vi "ScrimCode.vi"() -> ()   [LabVIEW 2017]
uses:
  050-Tests/Wall Following/XY.ctl
  040-typeDefs/LidarPoint.ctl
  <vilib>/myRIO/Common/Instrument Driver Framework/myRIO v1.0/Encoder/typedefs/Encoder Signal Mode.ctl
  <vilib>/myRIO/Instrument Drivers/Onboard IO/Encoder/typedefs/Encoder Reference.ctl
  <vilib>/myRIO/Common/Instrument Driver Framework/Utilities/typedefs/myRIO Generic Hardware Reference.ctl
  <vilib>/myRIO/Common/Instrument Driver Framework/Utilities/typedefs/Hardware Version Enum.ctl
  <vilib>/myRIO/Common/Instrument Driver Framework/Utilities/typedefs/myRIO v1.0 Reference.ctl
  <vilib>/myRIO/Common/Instrument Driver Framework/Utilities/typedefs/Generic FPGA Reference.ctl
  <vilib>/myRIO/Common/Instrument Driver Framework/myRIO v1.0/Encoder/typedefs/Encoder Channels Enum.ctl
  <vilib>/myRIO/Common/Instrument Driver Framework/myRIO v1.0/Encoder/typedefs/Encoder Configuration v1.0.ctl
  <vilib>/userdefined/High Color/nirio_resource_hc.ctl
  <vilib>/myRIO/Common/Instrument Driver Framework/Utilities/vis/Is FPGA Ref Available.vi
  <vilib>/myRIO/Common/Instrument Driver Framework/myRIO v1.0/Encoder/vis/myRIO v1.1 Open Encoder.vi
  <vilib>/myRIO/Instrument Drivers/Onboard IO/Encoder/vis/Read.vi
  <vilib>/myRIO/Common/Instrument Driver Framework/Utilities/vis/Validate Channels.vi
  <vilib>/myRIO/Common/Instrument Driver Framework/myRIO v1.0/Encoder/vis/myRIO v1.0 Reserve Encoder.vi
  <vilib>/myRIO/Common/Instrument Driver Framework/myRIO v1.0/Encoder/vis/myRIO v1.0 Build MUX Configuration Encoder.vi
  <vilib>/myRIO/Common/Instrument Driver Framework/myRIO v1.0/Resource Manager/vis/myRIO v1.0 Reserve Channel List.vi
  <vilib>/myRIO/Common/Instrument Driver Framework/myRIO v1.0/Resource Manager/vis/myRIO v1.0 Create Configuration List.vi
  <vilib>/myRIO/Common/Instrument Driver Framework/myRIO v1.0/Resource Manager/vis/myRIO v1.0 Reserve Channel.vi
  <vilib>/myRIO/Common/Instrument Driver Framework/myRIO v1.0/Resource Manager/vis/myRIO v1.0 Unreserve Channel.vi
  <vilib>/myRIO/Common/Instrument Driver Framework/myRIO v1.0/Resource Manager/vis/myRIO v1.0 Build Mutex Name.vi
  <vilib>/Utility/VariantDataType/GetNumericInfo.vi
  <vilib>/Utility/error.llb/Error Cluster From Error Code.vi
  <vilib>/myRIO/Common/Instrument Driver Framework/myRIO v1.0/myRIO v1.1 Open.vi
  <vilib>/myRIO/Common/Instrument Driver Framework/Utilities/vis/IO Manager.vi
  <vilib>/myRIO/Common/Instrument Driver Framework/Utilities/vis/Configuration Manager.vi
  <vilib>/myRIO/Common/Instrument Driver Framework/myRIO v1.0/Resource Manager/vis/myRIO v1.0 Configure IO.vi
  <vilib>/myRIO/Common/Instrument Driver Framework/myRIO v1.0/myRIO v1.0 Close.vi
  <vilib>/myRIO/Common/Instrument Driver Framework/myRIO v1.0/Encoder/vis/myRIO v1.0 Configure Encoder.vi
  <vilib>/myRIO/Common/Instrument Driver Framework/myRIO v1.0/Encoder/vis/myRIO v1.0 Read Encoder.vi
  <vilib>/addons/control/pid/pid.llb/PID (DBL).vi
  <vilib>/myRIO/Express VI/Onboard IO/Encoder/Encoder Express VI.xnode
  <vilib>/myRIO/Instrument Drivers/Onboard IO/Encoder/vis/myRIO Encoder Open.xnode
  <vilib>/myRIO/Common/Instrument Driver Framework/myRIO v1.0/Encoder/typedefs/Encoder Count Direction Enum.ctl
  <vilib>/addons/control/pid/NI_PID_pid.lvlib
  <vilib>/myRIO/Instrument Drivers/Onboard IO/Encoder/Encoder.lvlib
panel:
  out "XY Graph":cluster{dbl[], dbl[]}(graph)
  in  "Stop Lidar":bool
  out "LidarXY":T1=[{"X"=0.0, "Y"=-0.0}, {"X"=0.0, "Y"=-0.0}, {"X"=0.0, "Y"=-0.0}, {"X"=0.0, "Y"=-0.0}, {"X"=0.0, "Y"=-0.0}, {"X"=0.0, "Y"=-0.0}, {"X"=0.0, "Y"=-0.0}, {"X"=0.0, "Y"=-0.0}, {"X"=0.0, "Y"=-0.0}, {"X"=0.0, "Y"=-0.0}, {"X"=0.0, "Y"=-0.0}, {"X"=0.0, "Y"=-0.0}, {"X"=0.0, "Y"=-0.0}, {"X"=0.0, "Y"=-0.0}, {"X"=0.0, "Y"=-0.0}, {"X"=0.0, "Y"=-0.0}, {"X"=0.0, "Y"=-0.0}, {"X"=0.0, "Y"=-0.0}, {"X"=0.0, "Y"=-0.0}, {"X"=0.0, "Y"=-0.0}, {"X"=0.0, "Y"=-0.0}, {"X"=0.0, "Y"=-0.0}, {"X"=0.0, "Y"=-0.0}, {"X"=0.0, "Y"=-0.0}, {"X"=0.0, "Y"=-0.0}, {"X"=0.0, "Y"=-0.0}, {"X"=0.0, "Y"=-0.0}, {"X"=0.0, "Y"=-0.0}, {"X"=0.0, "Y"=-0.0}, {"X"=0.0, "Y"=-0.0}, {"X"=0.0, "Y"=-0.0}, {"X"=0.0, "Y"=-0.0}, {"X"=0.0, "Y"=-0.0}, {"X"=0.0, "Y"=-0.0}, {"X"=1175.808659612749, "Y"=-52.94332799957733}, {"X"=1168.1174194020048, "Y"=-45.41689652101715}, {"X"=1160.3783860600606, "Y"=-37.98685515608209}, {"X"=1168.5867974931368, "Y"=-31.07887907782929}, {"X"=1168.7554955939645, "Y"=-23.907980234770854}, {"X"=1168.8801907109664, "Y"=-16.736181269769418}, {"X"=1176.960610420781, "Y"=-9.629201313834}, {"X"=1176.9975381384256, "Y"=-2.4073255047001396}, {"X"=1193.9900103325547, "Y"=4.884181207324338}, {"X"=1195.9374604543593, "Y"=12.230726960306109}, {"X"=1201.8390977672932, "Y"=19.66680141503711}, {"X"=1204.6950410270608, "Y"=27.108266724527297}, {"X"=1207.5047999843382, "Y"=34.58551741384792}, {"X"=1227.2577678305224, "Y"=42.689241029135935}, {"X"=1235.9651999305015, "Y"=50.586802238878725}, {"X"=1235.6315384515906, "Y"=58.169589853765174}, {"X"=1239.245701676844, "Y"=65.96279917852931}, {"X"=1239.8158745447101, "Y"=73.62470527571115}, {"X"=1238.342923739107, "Y"=81.16528337460754}, {"X"=1238.819030299992, "Y"=88.83360944252911}, {"X"=1250.2144113728411, "Y"=97.36490946773479}, {"X"=1258.5618306768233, "Y"=105.78808233162614}, {"X"=1257.8890351355897, "Y"=113.50848111773375}, {"X"=1258.1642639033219, "Y"=121.3205878514131}, {"X"=1267.3439246949379, "Y"=130.059127087766}, {"X"=1296.3459493807188, "Y"=141.0786288712885}, {"X"=1298.4362471784139, "Y"=149.37306321166824}, {"X"=1302.4589077275016, "Y"=157.9392088155543}, {"X"=1325.2725844764723, "Y"=168.96324107643002}, {"X"=1341.0608866043438, "Y"=179.34519346771347}, {"X"=1362.713108150387, "Y"=190.75897062815193}, {"X"=0.0, "Y"=0.0}, {"X"=0.0, "Y"=0.0}, {"X"=0.0, "Y"=0.0}, {"X"=0.0, "Y"=0.0}, {"X"=2289.607457999501, "Y"=392.4623399423975}, {"X"=2281.2488327694173, "Y"=405.4537741693527}, {"X"=2278.718071315956, "Y"=419.44362131052713}, {"X"=2281.995608526178, "Y"=434.54003574727074}, {"X"=2280.2675453173724, "Y"=448.7270013853459}, {"X"=2286.2910941419436, "Y"=464.5019190996244}, {"X"=2285.355403024562, "Y"=478.9318133789431}, {"X"=6.842233824605003, "Y"=1.477780866512756}, {"X"=3685.935672545284, "Y"=819.7891301170949}, {"X"=3639.8946504738656, "Y"=833.0203679693163}, {"X"=3675.598054671661, "Y"=864.959502227648}, {"X"=3670.221570845151, "Y"=887.4962652895791}, {"X"=0.0, "Y"=0.0}, {"X"=0.0, "Y"=0.0}, {"X"=0.0, "Y"=0.0}, {"X"=0.0, "Y"=0.0}, {"X"=0.0, "Y"=0.0}, {"X"=0.0, "Y"=0.0}, {"X"=0.0, "Y"=0.0}, {"X"=0.0, "Y"=0.0}, {"X"=0.0, "Y"=0.0}, {"X"=0.0, "Y"=0.0}, {"X"=0.0, "Y"=0.0}, {"X"=0.0, "Y"=0.0}, {"X"=0.0, "Y"=0.0}, {"X"=0.0, "Y"=0.0}, {"X"=0.0, "Y"=0.0}, {"X"=0.0, "Y"=0.0}, {"X"=0.0, "Y"=0.0}, {"X"=600.7610289106608, "Y"=217.73191346746614}, {"X"=599.4137418485913, "Y"=221.4140151008296}, {"X"=598.0438871979312, "Y"=225.0877806216682}, {"X"=0.0, "Y"=0.0}, {"X"=0.0, "Y"=0.0}, {"X"=0.0, "Y"=0.0}, {"X"=0.0, "Y"=0.0}, {"X"=0.0, "Y"=0.0}, {"X"=0.0, "Y"=0.0}, {"X"=0.0, "Y"=0.0}, {"X"=0.0, "Y"=0.0}, {"X"=0.0, "Y"=0.0}, {"X"=0.0, "Y"=0.0}, {"X"=0.0, "Y"=0.0}, {"X"=0.0, "Y"=0.0}, {"X"=0.0, "Y"=0.0}, {"X"=0.0, "Y"=0.0}, {"X"=0.0, "Y"=0.0}, {"X"=0.0, "Y"=0.0}, {"X"=0.0, "Y"=0.0}, {"X"=0.0, "Y"=0.0}, {"X"=0.0, "Y"=0.0}, {"X"=0.0, "Y"=0.0}, {"X"=0.0, "Y"=0.0}, {"X"=0.0, "Y"=0.0}, {"X"=0.0, "Y"=0.0}, {"X"=0.0, "Y"=0.0}, {"X"=0.0, "Y"=0.0}, {"X"=0.0, "Y"=0.0}, {"X"=0.0, "Y"=0.0}, {"X"=0.0, "Y"=0.0}, {"X"=0.0, "Y"=0.0}, {"X"=0.0, "Y"=0.0}, {"X"=0.0, "Y"=0.0}, {"X"=0.0, "Y"=0.0}, {"X"=0.0, "Y"=0.0}, {"X"=0.0, "Y"=0.0}, {"X"=0.0, "Y"=0.0}, {"X"=0.0, "Y"=0.0}, {"X"=0.0, "Y"=0.0}, {"X"=0.0, "Y"=0.0}, {"X"=0.0, "Y"=0.0}, {"X"=0.0, "Y"=0.0}, {"X"=0.0, "Y"=0.0}, {"X"=0.0, "Y"=0.0}, {"X"=3374.8558314202755, "Y"=2428.849957722494}, {"X"=3359.889157542298, "Y"=2449.5119613975567}, {"X"=3344.7959857365563, "Y"=2470.0817423317426}, {"X"=3345.592165080973, "Y"=2502.53812457449}, {"X"=3335.7534158602557, "Y"=2527.246356922221}, {"X"=3324.9438491605665, "Y"=2551.319148975548}, {"X"=3334.493957734356, "Y"=2591.3083656394642}, {"X"=3326.3894492365894, "Y"=2617.9041678425706}, {"X"=3315.7377682709716, "Y"=2642.62805783588}, {"X"=3309.5767598797984, "Y"=2671.0879188943845}, {"X"=3293.1249706744984, "Y"=2691.344817655309}, {"X"=3276.5491971753336, "Y"=2711.500388805002}, {"X"=3267.514888429531, "Y"=2737.9765254456347}, {"X"=1899.455264930813, "Y"=1611.5677759643295}, {"X"=1862.223559000626, "Y"=1599.7338579598302}, {"X"=1835.0185160308536, "Y"=1596.036041517836}, {"X"=1824.440389608465, "Y"=1606.6045763551506}, {"X"=1814.5481046764007, "Y"=1617.7688882579248}, {"X"=1802.3605336758628, "Y"=1626.8621658418574}, {"X"=1792.344366158486, "Y"=1637.8906169521624}, {"X"=1793.271389539639, "Y"=1659.0439184839483}, {"X"=1813.7122206541214, "Y"=1698.726870526835}, {"X"=1812.6884124722617, "Y"=1718.768372785813}, {"X"=1817.2579527606933, "Y"=1744.4009095182257}, {"X"=1817.994824175701, "Y"=1766.6691312383205}, {"X"=1826.3679604567812, "Y"=1796.725931525712}, {"X"=1829.4801075764935, "Y"=1822.0116728445792}, {"X"=1820.378639790371, "Y"=1835.3328329747055}, {"X"=1844.7747536692077, "Y"=1882.8972643839902}, {"X"=1874.2179013509035, "Y"=1936.577459916286}, {"X"=1897.542044708991, "Y"=1984.905586813041}, {"X"=0.0, "Y"=0.0}, {"X"=0.0, "Y"=0.0}, {"X"=0.0, "Y"=0.0}, {"X"=0.0, "Y"=0.0}, {"X"=0.0, "Y"=0.0}, {"X"=0.0, "Y"=0.0}, {"X"=0.0, "Y"=0.0}, {"X"=0.0, "Y"=0.0}, {"X"=0.0, "Y"=0.0}, {"X"=0.0, "Y"=0.0}, {"X"=0.0, "Y"=0.0}, {"X"=0.0, "Y"=0.0}, {"X"=0.0, "Y"=0.0}, {"X"=0.0, "Y"=0.0}, {"X"=0.0, "Y"=0.0}, {"X"=0.0, "Y"=0.0}, {"X"=0.0, "Y"=0.0}, {"X"=0.0, "Y"=0.0}, {"X"=0.0, "Y"=0.0}, {"X"=1743.6379817840352, "Y"=2341.001407193105}, {"X"=1462.0647125166643, "Y"=1988.3135508298394}, {"X"=1449.8371269673896, "Y"=1997.2471818147462}, {"X"=1404.3537271482712, "Y"=1959.773356550384}, {"X"=1392.3023473319502, "Y"=1968.3534168471733}, {"X"=1383.633301868133, "Y"=1981.7789700068693}, {"X"=1371.4472882021594, "Y"=1990.2314779148037}, {"X"=1359.20964032093, "Y"=1998.6090547324775}, {"X"=1351.9362460939265, "Y"=2014.3843691057232}, {"X"=1353.9070398167903, "Y"=2044.3188908618283}, {"X"=1344.0730393692736, "Y"=2056.773362536729}, {"X"=1331.427613472165, "Y"=2064.981721489034}, {"X"=1335.9072436035742, "Y"=2100.1125770985473}, {"X"=1341.5998483880717, "Y"=2137.9162394268637}, {"X"=1344.7728116096719, "Y"=2172.4665901125886}, {"X"=1342.8817524476133, "Y"=2199.453931989308}, {"X"=1347.9316929777974, "Y"=2238.492606882142}, {"X"=1334.681775935609, "Y"=2247.5810456989907}, {"X"=1391.1030672198049, "Y"=2375.6770101113602}, {"X"=1379.5000000000002, "Y"=2389.364089041266}, {"X"=1385.0949158492374, "Y"=2433.4157215914825}, {"X"=1373.5630278668962, "Y"=2447.9733675996404}, {"X"=1361.9045108896655, "Y"=2462.480883828011}, {"X"=1355.8627003263439, "Y"=2487.4736858635824}, {"X"=1349.5651164388382, "Y"=2512.484427114211}, {"X"=1335.5267522358927, "Y"=2523.369432735177}, {"X"=1969.6248133756371, "Y"=3777.324197700667}, {"X"=1969.2557039671133, "Y"=3833.8142850681993}, {"X"=1962.397971406475, "Y"=3878.8404455223153}, {"X"=1938.5609122730393, "Y"=3890.808475035378}, {"X"=1915.9722275738832, "Y"=3905.323344252761}, {"X"=0.0, "Y"=0.0}, {"X"=0.0, "Y"=0.0}, {"X"=0.0, "Y"=0.0}, {"X"=0.0, "Y"=0.0}, {"X"=0.0, "Y"=0.0}, {"X"=0.0, "Y"=0.0}, {"X"=0.0, "Y"=0.0}, {"X"=0.0, "Y"=0.0}, {"X"=0.0, "Y"=0.0}, {"X"=58.83955402796909, "Y"=141.23351897403714}, {"X"=53.04614074023745, "Y"=129.5612092895359}, {"X"=52.25016952642336, "Y"=129.88425533705006}, {"X"=50.34968331347441, "Y"=127.41235964470965}, {"X"=49.56694795325839, "Y"=127.71890099197915}, {"X"=51.274875074943694, "Y"=134.5618340617016}, {"X"=50.44825394792947, "Y"=134.87391769206238}, {"X"=49.27515199021851, "Y"=134.2421669831833}, {"X"=48.78934484248565, "Y"=135.48283961388253}, {"X"=47.62408377020564, "Y"=134.83674070908282}, {"X"=46.79584457282841, "Y"=135.12641833007964}, {"X"=44.358646211836316, "Y"=130.67635787032458}, {"X"=45.13411191584662, "Y"=135.69050055758447}, {"X"=42.7517061587144, "Y"=131.2108670062009}, {"X"=41.94580662526205, "Y"=131.47071653625426}, {"X"=40.24401638076991, "Y"=128.86201591448244}, {"X"=38.28361110853757, "Y"=125.28114431346107}, {"X"=36.655076426411945, "Y"=122.63933044571753}, {"X"=35.90188561989253, "Y"=122.86193311573831}, {"X"=34.598165891301484, "Y"=121.1567865080532}, {"X"=35.197527608421304, "Y"=126.18293882397263}, {"X"=34.42262106759573, "Y"=126.39653143514941}, {"X"=33.646418534542704, "Y"=126.60536528835728}, {"X"=31.865317195204643, "Y"=122.93738878001678}, {"X"=31.355351385691893, "Y"=124.10012868438046}, {"X"=30.354286922264357, "Y"=123.31916828068883}, {"X"=29.36399573459602, "Y"=122.53063190279657}, {"X"=28.611609142331027, "Y"=122.70849938894403}, {"X"=27.637048947572616, "Y"=121.90649500936969}, {"X"=26.88852449657622, "Y"=122.07377789843738}, {"X"=26.138987707829987, "Y"=122.2364647787636}, {"X"=24.169820394523793, "Y"=116.5196111480658}, {"X"=23.454414511116422, "Y"=116.6657209292461}, {"X"=22.547048896693994, "Y"=115.8258632001078}, {"X"=22.39108108970486, "Y"=118.91021607765357}, {"X"=21.30300649191931, "Y"=117.07767470532221}, {"X"=20.93018381331909, "Y"=119.17603536592698}, {"X"=20.19853940257479, "Y"=119.30221710430462}, {"X"=19.948765962822694, "Y"=122.38483050019119}, {"X"=19.197451230185493, "Y"=122.50492996718397}, {"X"=18.44541372435992, "Y"=122.62041719280356}, {"X"=17.69268175913302, "Y"=122.73128782902118}, {"X"=16.939283674437824, "Y"=122.83753770162004}, {"X"=16.18524783528641, "Y"=122.93916281035249}, {"X"=15.555042974497924, "Y"=124.02838642045425}, {"X"=14.793726282913141, "Y"=124.12149557053462}, {"X"=14.031852615895252, "Y"=124.20993161646051}, {"X"=13.37560626281767, "Y"=125.28804075849406}, {"X"=12.606601504797023, "Y"=125.3677534236745}, {"X"=11.367395047285386, "Y"=120.4648593152333}, {"X"=10.62802257825117, "Y"=120.53234062307172}, {"X"=9.643086747772859, "Y"=117.60531823848328}, {"X"=8.921292552551547, "Y"=117.66227321954896}, {"X"=8.199162475707965, "Y"=117.71479828253092}, {"X"=7.856896096812613, "Y"=123.75083508293547}, {"X"=7.612563199246648, "Y"=132.7819599250496}, {"X"=6.7976851053069876, "Y"=132.82617015185332}, {"X"=6.027532669450633, "Y"=133.86436736457804}, {"X"=5.594553549210016, "Y"=143.89128177407073}, {"X"=0.0, "Y"=0.0}, {"X"=0.0, "Y"=0.0}, {"X"=0.0, "Y"=0.0}, {"X"=0.0, "Y"=0.0}, {"X"=0.0, "Y"=0.0}, {"X"=0.0, "Y"=0.0}, {"X"=-0.0, "Y"=0.0}, {"X"=-0.0, "Y"=0.0}, {"X"=-0.0, "Y"=0.0}, {"X"=-0.0, "Y"=0.0}, {"X"=-0.0, "Y"=0.0}, {"X"=-0.0, "Y"=0.0}, {"X"=-0.0, "Y"=0.0}, {"X"=-14.389567093979142, "Y"=305.6614800050014}, {"X"=-16.264799797445626, "Y"=305.5674332901807}, {"X"=-18.020861838821443, "Y"=303.4653992444379}, {"X"=-19.5555356398128, "Y"=298.35981804834245}, {"X"=-20.81367177759742, "Y"=290.25470033598845}, {"X"=-22.594249326244693, "Y"=290.1215260841282}, {"X"=-24.373976214175155, "Y"=289.97742892078827}, {"X"=-26.871762354871255, "Y"=297.7900407803178}, {"X"=-28.890424796895044, "Y"=299.61031917318024}, {"X"=-31.238691435523062, "Y"=304.40128803504786}, {"X"=-33.10587456642204, "Y"=304.20388075958584}, {"X"=-34.97181127985504, "Y"=303.99502037994995}, {"X"=-36.23452885173925, "Y"=298.8110756295564}, {"X"=-37.434969579807884, "Y"=293.6232672193382}, {"X"=-38.83824219219518, "Y"=290.41451572437006}, {"X"=-39.23313131378416, "Y"=280.26730349313914}, {"X"=-40.95208060633797, "Y"=280.02129757218825}, {"X"=-42.21716134748016, "Y"=276.79904495456776}, {"X"=-43.91477363218576, "Y"=276.53479465852735}, {"X"=-45.61073255048484, "Y"=276.26013298376614}, {"X"=-47.30497425048268, "Y"=275.9750702711409}, {"X"=-47.94748991040257, "Y"=269.7721968833924}, {"X"=-49.6018783940805, "Y"=269.4729182307173}, {"X"=-49.383800877003665, "Y"=259.34000888975936}, {"X"=-50.974151620366335, "Y"=259.0321135816637}, {"X"=-52.562583215731195, "Y"=258.7144658608972}, {"X"=-52.9183759536477, "Y"=252.51464410292803}, {"X"=-50.24454946143372, "Y"=232.6359500365701}, {"X"=-50.58550511580592, "Y"=227.442534878986}, {"X"=-51.08775154391361, "Y"=223.22867567180376}, {"X"=-52.456495235733954, "Y"=222.9110049046108}, {"X"=-51.94297527250979, "Y"=214.80904850550277}, {"X"=-53.260041003903865, "Y"=214.48628868126391}, {"X"=-54.5751015248568, "Y"=214.15545356948437}, {"X"=-55.12944523371112, "Y"=210.91406844547674}, {"X"=-56.42255183234955, "Y"=210.5718301310169}, {"X"=-58.772498083229195, "Y"=214.0789421429787}, {"X"=-59.002343593312666, "Y"=209.86358295449136}, {"X"=-60.56548636017391, "Y"=210.4585989261441}, {"X"=-62.420588118610965, "Y"=212.00158060478398}, {"X"=-63.14357664472082, "Y"=209.69952009604665}, {"X"=-62.958096488218466, "Y"=204.52940641037458}, {"X"=-63.01165810578052, "Y"=200.32356562012424}, {"X"=-62.71011911979348, "Y"=195.17284893135445}, {"X"=-52.683892407409445, "Y"=160.57835308909014}, {"X"=-45.72910940568647, "Y"=136.5461407472315}, {"X"=-42.03882216538083, "Y"=123.01519187054697}, {"X"=-40.81778377043683, "Y"=117.08931859085125}, {"X"=-40.53057173149517, "Y"=114.00996778842683}, {"X"=-41.22936076613992, "Y"=113.75913067009384}, {"X"=-40.54059431423641, "Y"=109.75181188777023}, {"X"=-37.69075512757198, "Y"=100.14193416303385}, {"X"=-36.87256085543507, "Y"=96.173875121897}, {"X"=-35.643435896144865, "Y"=91.2882548716833}, {"X"=-36.57231645821402, "Y"=91.99709598068979}, {"X"=-37.13611156368677, "Y"=91.77096064621645}, {"X"=-37.69850851554857, "Y"=91.54137018694395}, {"X"=-38.25948613987204, "Y"=91.30833324682331}, {"X"=-41.171691395934374, "Y"=96.59136518135533}, {"X"=-42.956835248917194, "Y"=99.08940561632906}, {"X"=-43.56402776144836, "Y"=98.82396210029101}, {"X"=-43.351624925679815, "Y"=96.72970906760331}, {"X"=-43.94433118057689, "Y"=96.46188758826865}, {"X"=-41.594367100641534, "Y"=89.83823587703105}, {"X"=-42.144821150860494, "Y"=89.58132645904493}, {"X"=-42.69368847238343, "Y"=89.3210443547492}, {"X"=-43.24094840066599, "Y"=89.05739936361796}, {"X"=-43.786580331681115, "Y"=88.79040141173614}, {"X"=-44.33056372269506, "Y"=88.5200605514257}, {"X"=-44.87287809304058, "Y"=88.24638696086723}, {"X"=-48.624558794324656, "Y"=94.1894488892321}, {"X"=-49.201579044298484, "Y"=93.88932111559679}, {"X"=-53.5334824964135, "Y"=100.64872702526439}, {"X"=-56.05004525698034, "Y"=103.83829942121768}, {"X"=-57.64691182182825, "Y"=105.24653703284663}, {"X"=-0.0, "Y"=0.0}, {"X"=-0.0, "Y"=0.0}, {"X"=-0.0, "Y"=0.0}]
  out "Numeric":i32=3
  out "latest notification":bool
  in  "Finish SZone":bool
  in  "angle\n 2":dbl(slide) scale=-90.0..90.0
  in  "Min Speed 2":dbl=1.0
  in  "Max Speed 2":dbl=3.0
  out "PID B 2":T3(graph)={"Setpoint"=1.4519657872720528, "output"=0.11191211724832612, "dx/dt"=1.0}
  out "PID A 2":T3(graph)={"Setpoint"=2.286351969737293, "output"=0.16194563982689175, "dx/dt"=1.8520000000025902}
  out "OUTPUT A 2":dbl(slide)=1.8520000000025902 scale=-10.0..10.0
  out "OUTPUT B 2":dbl(slide)=1.0 scale=-10.0..10.0
  in  "PID gains 2":T4={"proportional gain (Kc)"=0.04, "integral time (Ti, min)"=0.1, "derivative time (Td, min)"=0.0} {"derivative time (Td, min)" format="%.3f"; "integral time (Ti, min)" format="%.3f"; "proportional gain (Kc)" format="%.3f"}
  out "XY Graph 2":cluster{"X":dbl, "Y":dbl}[](graph)=[{"X"=2749.19090547731, "Y"=10902.248088916496}, {"X"=2748.940240600598, "Y"=10902.411520010117}]
  in  "speed 2":dbl(slide)=1.8691588785046729 scale=0.0..10.0
  out "Waveform Chart 3":dbl(graph)=-56.89603549696165
  in  "Initial X, Y, BEARING 2":cluster{dbl, dbl, dbl}
  out "Final X, Y, BEARING 2":cluster{dbl, dbl, dbl}={280.04170712542475, 2538.178279000119, -2.5725196254764082}
  in  "stop 2":bool
  in  "stop":bool
  in  "Boolean":bool
  in  "START CODE":bool
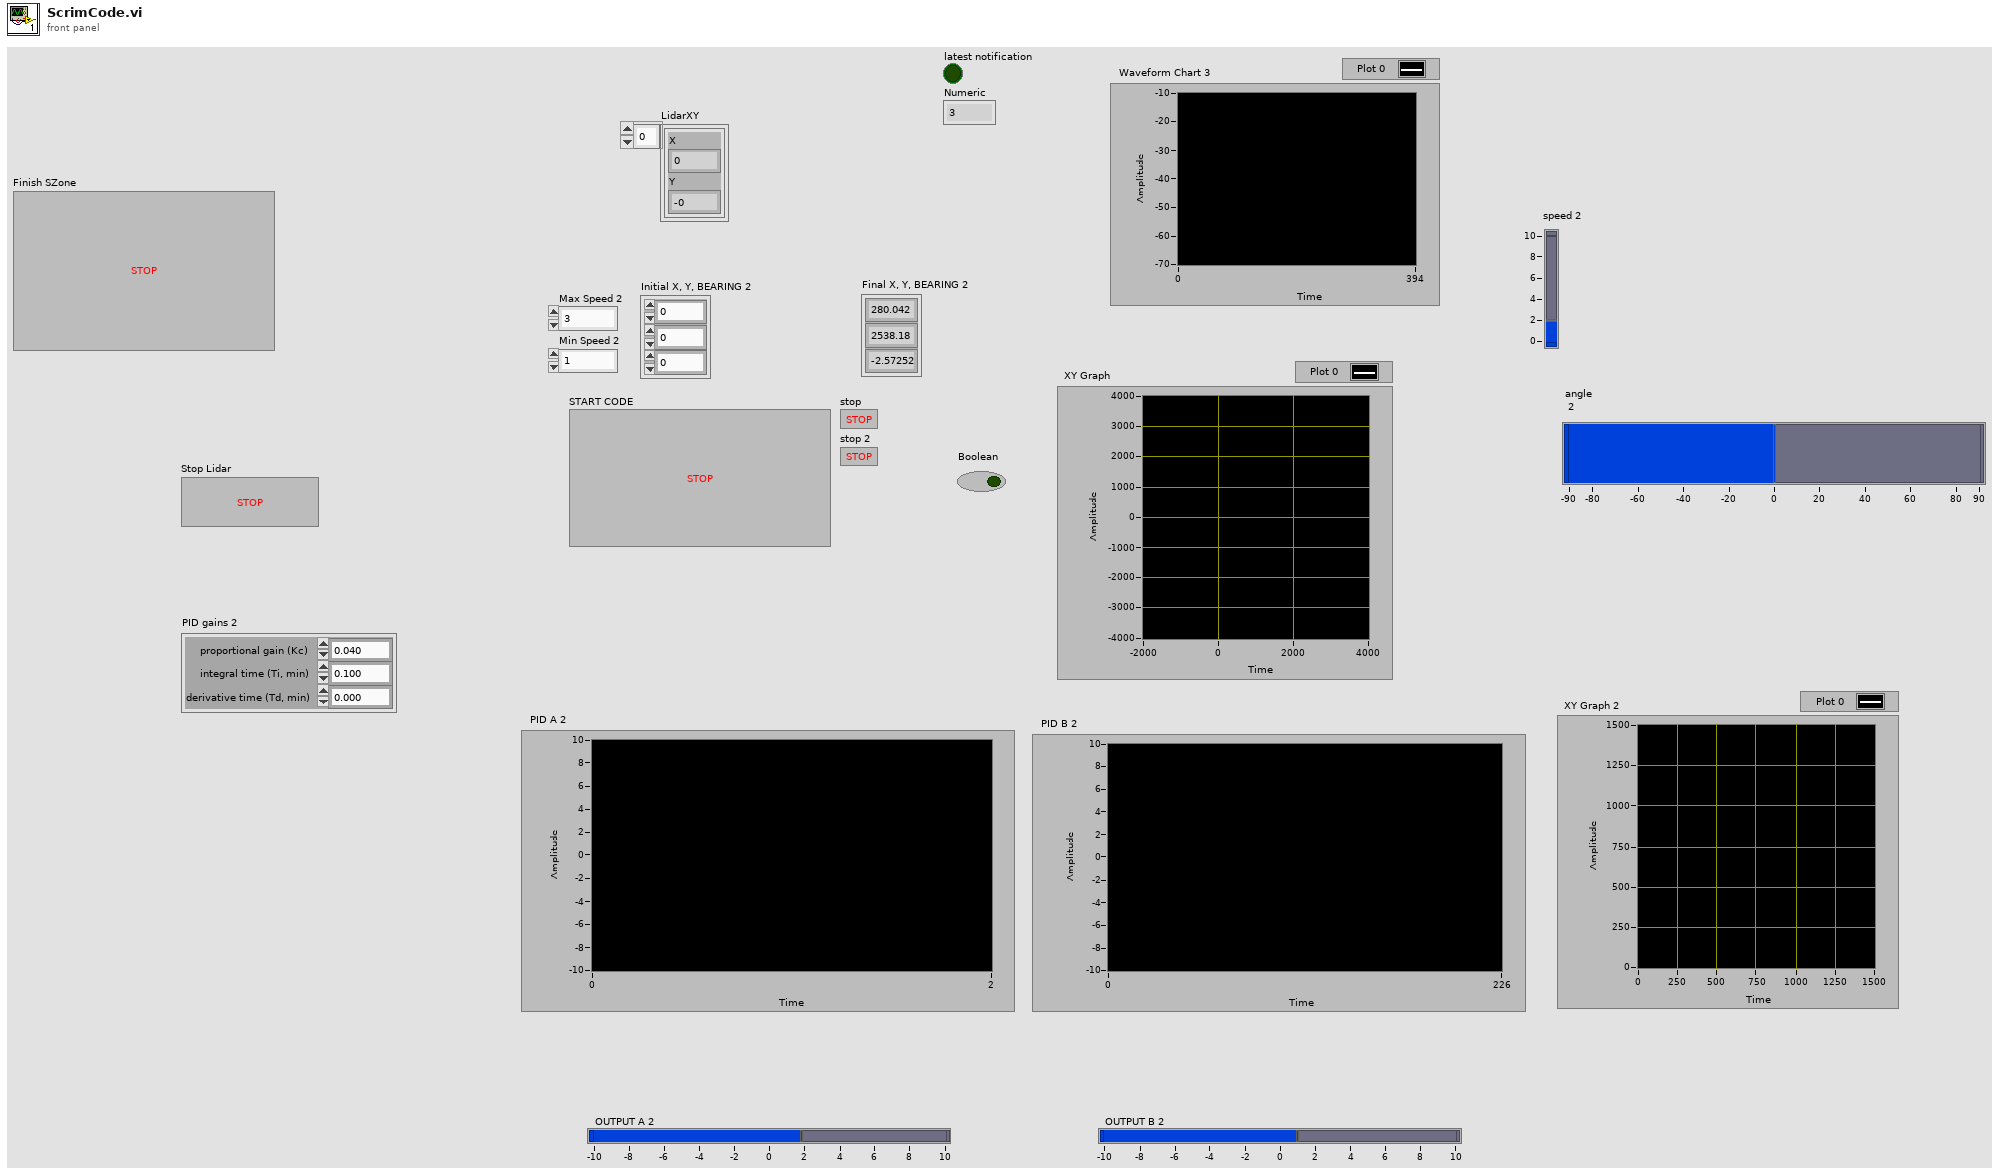
[diagram p1: front panel]
types:
  T1 = typedef "XY.ctl" = T2[]
  T2 = typedef "LidarPoint.ctl" = cluster{"X":dbl, "Y":dbl}
  T3 = cluster{"Setpoint":dbl, "output":dbl, "dx/dt":dbl}
  T4 = cluster{"proportional gain (Kc)":dbl, "integral time (Ti, min)":dbl, "derivative time (Td, min)":dbl}
  T5 = cluster{"Strength":dbl, "Distance from Wall":dbl}
  T6 = typedef "Encoder.lvlib/Encoder Reference.ctl" = cluster{"myRIO Reference":T7, "Encoder Channels Enum":T11}
  T7 = typedef "myRIO Generic Hardware Reference.ctl" = cluster{"myRIO Model":T8, "myRIO Hardware Reference":T9}
  T8 = typedef "Hardware Version Enum.ctl" = enum16{"Unknown", "myRIO-1900", "myRIO-1950", "roboRIO", "NI ELVIS RIO CM"}
  T9 = typedef "myRIO v1.0 Reference.ctl" = cluster{"Generic FPGA Reference":T10, "Allow multiple opens":bool}
  T10 = typedef "Generic FPGA Reference.ctl" = refnum<k20>
  T11 = typedef "Encoder Channels Enum.ctl" = enum16{"Not Connected", "C/ENC0", "C/ENC1", "A/ENC", "B/ENC", "DIO/ENC0", "DIO/ENC1", "DIO/ENC2", "DIO/ENC3", "DIO/ENC4"}
  T12 = typedef "Encoder Signal Mode.ctl" = enum16{"Quadrature phase signal", "Step and direction signal"}
  T13 = typedef "nirio_resource_hc.ctl" = tag
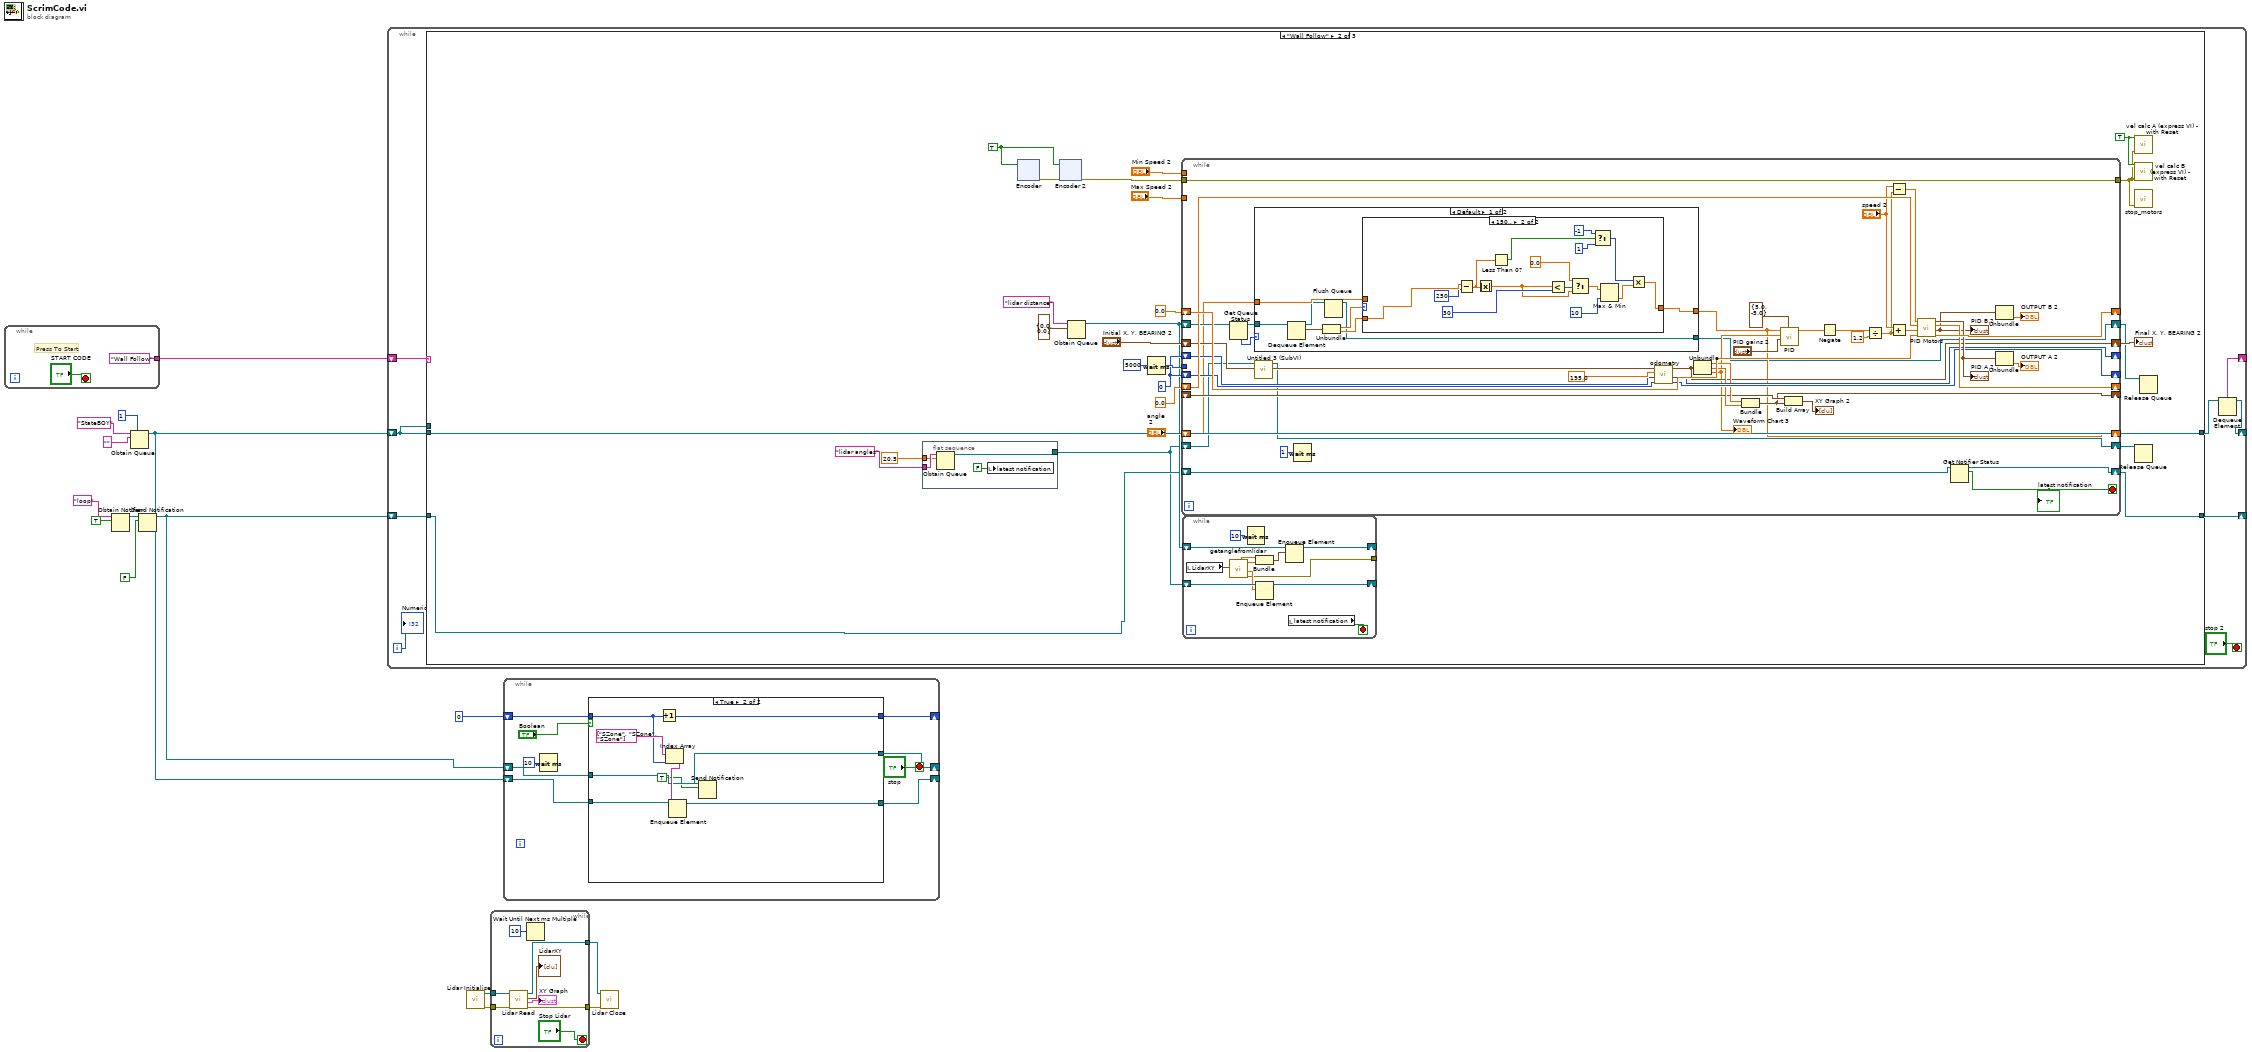
[diagram p0: block diagram]
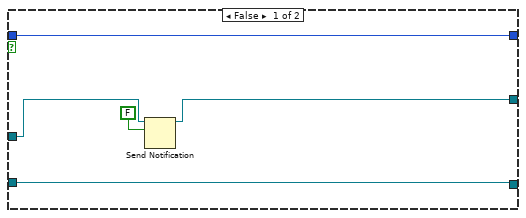
[diagram p2: hidden frame]
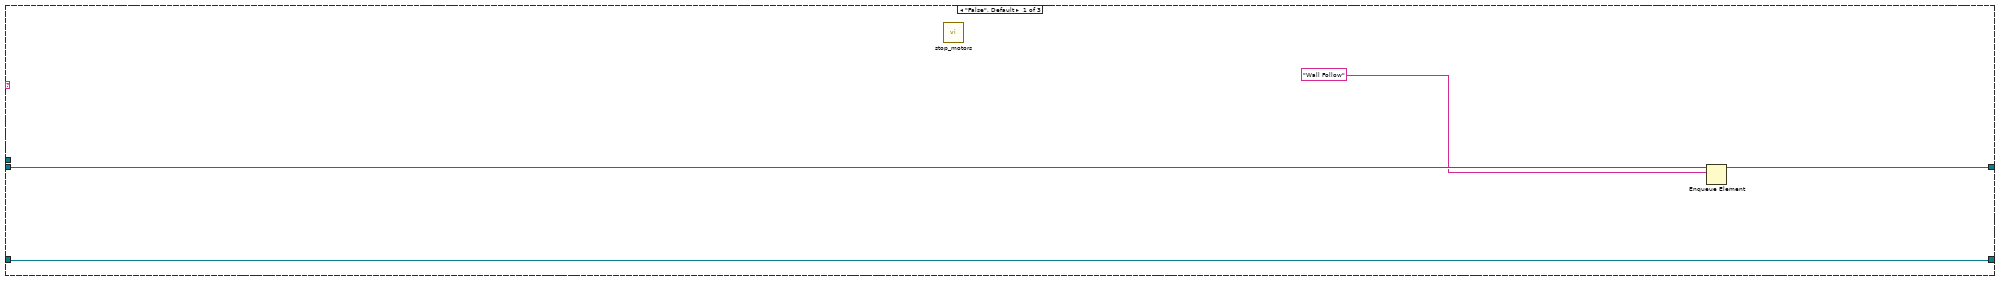
[diagram p3: hidden frame]
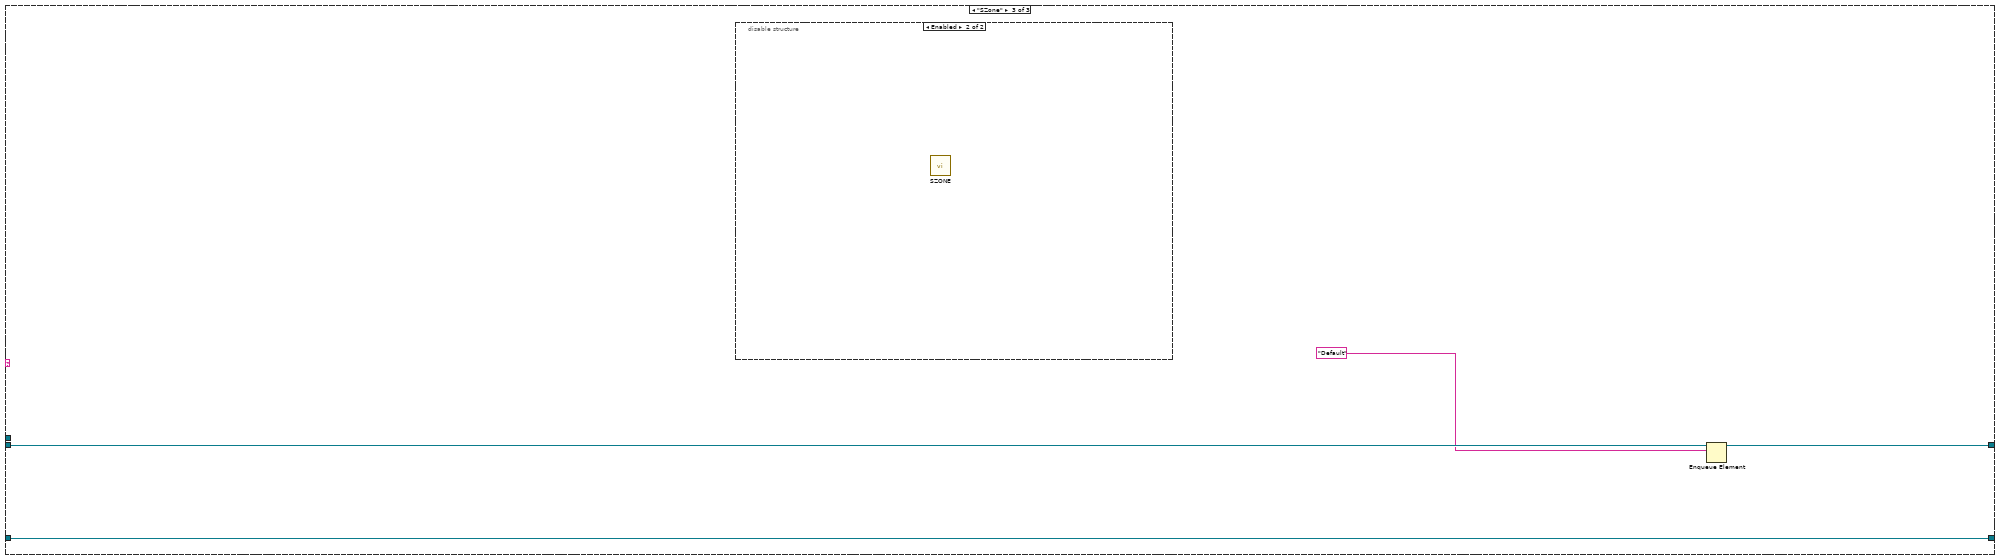
[diagram p6: hidden frame]
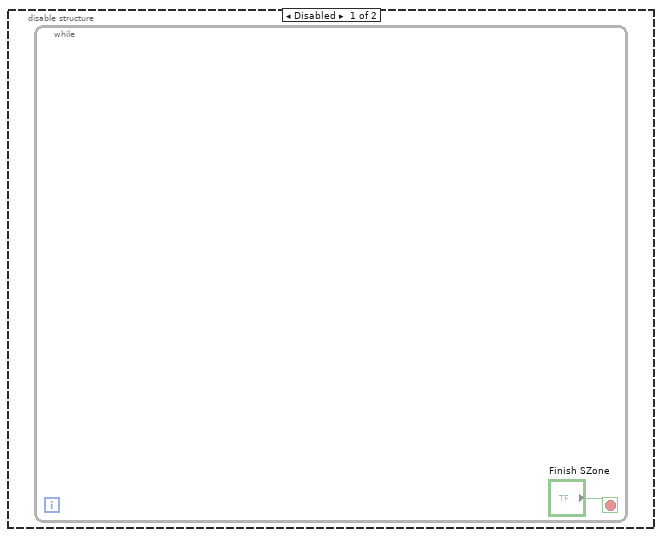
[diagram p7: hidden frame]
diagram:
  n1 = while {
    tunnel: ["Wall Follow"] -> w15
    stop <- "START CODE" stop-if-true
    # "Press To Start"
  }
  n2 = Obtain Notifier(name (unnamed)="loop", notification data type=TRUE) -> (notifier out=w8:refnum<notifier>)  [unwired: 2 in, 2 out]
  n3 = Obtain Queue(max queue size (-1, unlimited)=1, name (unnamed)="StateBOY", element data type="") -> (queue out=w13:refnum<queue>)  [unwired: 2 in, 2 out]
  n4 = Send Notification(notification=FALSE, notifier=w8) -> (notifier out=w5:refnum<notifier>)  [unwired: 1 in, 1 out]
  n5 = while {
    shift-right: [w18] -> _
    shift-left: w13 -> [w23]
    shift-right: [w24] -> _
    shift-left: w15 -> [w26]
    shift-right: [w20] -> _
    shift-left: w5 -> [w21]
    i -> [w19]
    stop <- "stop 2" stop-if-true
    n6 = case shown="\"Wall Follow\"" w26 {
      tunnel: [w29 w56 w237] -> w25
      tunnel: w23 -> [w30 w56 w238]
      tunnel: w23 -> [_ _ _]
      tunnel: w21 -> [w27 w34 w235]
      tunnel: [w27 w37 w235] -> w20
      frame "False", Default {
        n7 = call "stop_motors.vi"() -> ()  [unwired: 5 in, 1 out]
        n8 = Enqueue Element(queue=w30, element="Wall Follow") -> (queue out=w29:refnum<queue>)  [unwired: 2 in, 2 out]
      }
      frame "Wall Follow" {
        w43 = TRUE ("Reinitialise")
        w45 = TRUE
        w49 = 0 ("ENCA OUT")
        n9 = flat-sequence {
          tunnel: [w57] -> w33
          tunnel: "lidar angles" ("name (unnamed)") -> [w59]
          tunnel: 20.5 -> [w58]
          frame #0 {
            n10 = Obtain Queue(name (unnamed)=w59, element data type=w58) -> (queue out=w57:refnum<queue>)  [unwired: 3 in, 2 out]
            n11 = local write "latest notification"(FALSE ("latest notification")) -> ()
          }
        }
        n12 = xnode "Encoder"("Reset Counter"=w45) -> ("error out"=w46:errorcluster)  [unwired: 1 in, 3 out]
        n13 = xnode "Encoder 2"("error in (no error)"=w46, "Reset Counter"=w45) -> ("error out"=w44:errorcluster)  [unwired: 3 out]
        n14 = Obtain Queue(name (unnamed)="lidar distance", element data type=T5 {"Strength"=0.0, "Distance from Wall"=0.0} ("output cluster")) -> (queue out=w39:refnum<queue>)  [unwired: 3 in, 2 out]
        n15 = Wait (ms)(milliseconds to wait=u32 5000) -> (millisecond timer value=w53:u32)
        n16 = while {
          tunnel: w44 -> [w202]
          shift-right: [w204] -> _
          shift-left: 0.0 ("output A") -> [w205]
          shift-right: [w207] -> _
          shift-left: 0.0 ("output B") -> [w206]
          tunnel: [w202] -> w42
          shift-right: [w194] -> _
          shift-left: w49 -> [w196]
          shift-right: [w193] -> _
          shift-left: w49 -> [w195]
          shift-right: [w182] -> w55
          shift-left: "Initial X, Y, BEARING 2" -> [w186]
          shift-right: [w189] -> _
          shift-left: _ -> [w190]
          tunnel: "Max Speed 2" -> [_]
          tunnel: "Min Speed 2" -> [_]
          tunnel: w53 -> [_]
          shift-right: [w183] -> w35
          shift-left: w33 -> [w184]
          shift-right: [w170] -> _
          shift-left: "angle\n 2" -> [w171]
          shift-right: [w168] -> w36
          shift-left: w39 -> [w173]
          shift-right: [w167] -> w37
          shift-left: w34 -> [w166]
          stop <- w165 stop-if-true
          n17 = Get Queue Status(queue=w173) -> (queue out=w169:refnum<queue>, # elements in queue=w172:i32)  [unwired: 2 in, 6 out]
          n18 = case shown="Default" w172 {
            tunnel: w171 -> [w212 w234]
            tunnel: [w211 w234] -> w170
            tunnel: w169 -> [w216 w233]
            tunnel: [w209 w233] -> w168
            frame Default {
              n19 = Dequeue Element(queue=w216) -> (queue out=w210:refnum<queue>, element=w215:T5)  [unwired: 2 in, 2 out]
              n20 = Unbundle(w215) -> ("Strength"=w214:dbl, "Distance from Wall"=w213:dbl)
              n21 = Flush Queue(queue=w210) -> (queue out=w209:refnum<queue>)  [unwired: 1 in, 2 out]
              n22 = case shown="150.." w214 {
                tunnel: w213 -> [_ w232]
                tunnel: w212 -> [w217 _]
                tunnel: [w217 w218] -> w211
                frame 0, Default {
                }
                frame 150.. {
                  n23 = Subtract(x=w232, y=250) -> (x-y=w227:dbl)
                  n24 = Absolute Value(x=w227) -> (abs(x)=w223:dbl)
                  n25 = Less Than 0?(x=w227) -> (x < 0?=w226:bool)
                  n26 = Less?(x=w223, y=30) -> (x < y?=w229:bool)
                  n27 = Select(t=0.0, s=w229, f=w223) -> (s? t:f=w222:dbl)
                  n28 = Select(t=-1, s=w226, f=1) -> (s? t:f=w220:i32)
                  n29 = Max & Min(x=w222, y=10) -> (min(x,y)=w219:dbl)  [unwired: 1 out]
                  n30 = Multiply(x=w220, y=w219) -> (x*y=w218:dbl)
                }
              }
            }
            frame 0 {
            }
          }
          n31 = call "Untitled 3 (SubVI).vi"("X, Y, BEARING in"=w186, "Queue in"=w184) -> ("X, Y, BEARING out"=w185:cluster{dbl, dbl, dbl}, "Queue out"=w183:refnum<queue>)  [unwired: 8 in]
          n32 = Wait (ms)(milliseconds to wait=1 ("ENCB OUT")) -> ()  [unwired: 1 out]
          n33 = call "odometry.vi"("ENCB in"=w195, "ENCA in"=w196, "wheelbase"=195.0, "Position"=w185) -> ("ENCB OUT"=w193:i32, "ENCA OUT"=w194:i32, "X, Y, BEARING"=w182:cluster{dbl, dbl, dbl})  [unwired: 4 in]
          n34 = Unbundle(w182) -> (w191:dbl, w192:dbl, w178:dbl)
          "Waveform Chart 3" <- w178
          n35 = Bundle(w191, w192) -> (w189:cluster{dbl, dbl})  [unwired: 1 in]
          n36 = call-poly <vilib>:"PID.vi"("output range"=cluster{"output high":dbl, "output low":dbl} {"output high"=5.0, "output low"=-5.0}, "PID gains"="PID gains 2", "process variable"=w178, "setpoint"=w170) -> ("output"=w175:dbl)  [unwired: 6 in, 1 out]
          n37 = Build Array(w190, w189) -> (→"XY Graph 2":cluster{dbl, dbl}[])
          n38 = Negate(x=w175) -> (-x=w174:dbl)
          n39 = Divide(x=w174, y=1.2) -> (x/y=w177:dbl)
          n40 = Subtract(x="speed 2", y=w177) -> (x-y=w180:dbl)
          n41 = Add(x="speed 2", y=w177) -> (x+y=w179:dbl)
          n42 = call "PID Motors.vi"("input B"=w206, "Speed B"=w179, "input A"=w205, "Speed A"=w180) -> ("output B"=w207:dbl, "Speed B0"=w200:T3, "output A"=w204:dbl, "Speed A0"=w201:T3)
          "PID B 2" <- w200
          "PID A 2" <- w201
          n43 = Get Notifier Status(notifier=w166) -> (notifier out=w167:refnum<notifier>, current notification=w165:bool)  [unwired: 1 in, 3 out]
          "latest notification" <- w165
          n44 = Unbundle(w200) -> ("dx/dt"=→"OUTPUT B 2":dbl)  [unwired: 2 out]
          n45 = Unbundle(w201) -> ("dx/dt"=→"OUTPUT A 2":dbl)  [unwired: 2 out]
        }
        "Final X, Y, BEARING 2" <- w55
        n46 = while {
          shift-right: [w70] -> _
          shift-left: w33 -> [w72]
          shift-right: [w65] -> _
          shift-left: w39 -> [w66]
          tunnel: [w62] -> _
          stop <- w63 stop-if-true
          n47 = local read "LidarXY"() -> (w61:T1)
          n48 = call "getanglefromlidar.vi"("XY Array"=w61) -> ("error constant"=w62:errorcluster, "Angle From WALL"=w71:dbl, "Distance from Wall"=w67:dbl, "Strength"=w68:dbl)  [unwired: 5 in, 2 out]
          n49 = Wait (ms)(milliseconds to wait=10 ("ENCB OUT")) -> ()  [unwired: 1 out]
          n50 = Bundle("Strength"=w68, "Distance from Wall"=w67) -> (w64:T5)  [unwired: 1 in]
          n51 = Enqueue Element(queue=w72, element=w71) -> (queue out=w70:refnum<queue>)  [unwired: 2 in, 2 out]
          n52 = Enqueue Element(queue=w66, element=w64) -> (queue out=w65:refnum<queue>)  [unwired: 2 in, 2 out]
          n53 = local read "latest notification"() -> (w63:bool)
        }
        n54 = Release Queue(queue=w35) -> ()  [unwired: 2 in, 3 out]
        n55 = call "vel calc A (express VI) - with Reset.vi"("error in"=w42, "Reinitialise"=w43) -> ()  [unwired: 5 in, 5 out]
        n56 = call "vel calc B (express VI) - with Reset.vi"("error in"=w42, "Reinitialise"=w43) -> ()  [unwired: 5 in, 5 out]
        n57 = call "stop_motors.vi"("error in (no error)"=w42) -> ()  [unwired: 4 in, 1 out]
        n58 = Release Queue(queue=w36) -> ()  [unwired: 2 in, 3 out]
      }
      frame "SZone" {
        n59 = disable-structure shown="Enabled" {
          frame Disabled {
            n60 = while {
              stop <- "Finish SZone" stop-if-true
            }
          }
          frame Enabled {
            n61 = call "SZONE.vi"() -> ()  [unwired: 12 in]
          }
        }
        n62 = Enqueue Element(queue=w238, element="Default") -> (queue out=w237:refnum<queue>)  [unwired: 2 in, 2 out]
      }
    }
    n63 = Dequeue Element(queue=w25) -> (queue out=w18:refnum<queue>, element=w24:string)  [unwired: 2 in, 2 out]
    "Numeric" <- w19
  }
  n64 = call "Lidar Initialise.vi"() -> ("error out"=w3:errorcluster, "VISA resource name out"=w4:refnum<visa-resource-name>)  [unwired: 10 in]
  n65 = while {
    tunnel: w4 -> [w247]
    tunnel: w3 -> [w246]
    tunnel: [w245] -> w2
    tunnel: [w244] -> w1
    stop <- "Stop Lidar" stop-if-true
    n66 = call "Lidar Read.vi"("error in (no error)"=w246, "VISA resource name"=w247) -> ("error out"=w244:errorcluster, "Visual Out"=→"XY Graph":cluster{dbl[], dbl[]}, "XY Array"=→"LidarXY":T1, "VISA resource name out"=w245:refnum<visa-resource-name>)  [unwired: 2 in, 3 out]
    n67 = Wait Until Next ms Multiple(millisecond multiple=u32 10) -> ()  [unwired: 1 out]
  }
  n68 = while {
    shift-right: [w254] -> _
    shift-left: 0 -> [w255]
    shift-right: [w252] -> _
    shift-left: w13 -> [w253]
    shift-right: [w248] -> _
    shift-left: w5 -> [w249]
    stop <- "stop" stop-if-true
    n69 = Wait (ms)(milliseconds to wait=u32 10) -> ()  [unwired: 1 out]
    n70 = case shown="True" "Boolean" {
      tunnel: w255 -> [w261 w265]
      tunnel: [w261 w270] -> w254
      tunnel: w253 -> [w260 w269]
      tunnel: [w260 w268] -> w252
      tunnel: w249 -> [w259 w264]
      tunnel: [w257 w263] -> w248
      frame False {
        n71 = Send Notification(notification=FALSE, notifier=w259) -> (notifier out=w257:refnum<notifier>)  [unwired: 1 in, 1 out]
      }
      frame True {
        n72 = Increment(x=w265) -> (x+1=w270:i32)
        n73 = Index Array(array=string[] ["SZone", "SZone", "SZone"] ("Array"), index=w265) -> (element=w266:string)
        n74 = Enqueue Element(queue=w269, element=w266) -> (queue out=w268:refnum<queue>)  [unwired: 2 in, 2 out]
        n75 = Send Notification(notification=TRUE, notifier=w264) -> (notifier out=w263:refnum<notifier>)  [unwired: 1 in, 1 out]
      }
    }
  }
  n76 = call "Lidar Close.vi"("error in (no error)"=w1, "VISA resource name"=w2) -> ()  [unwired: 9 in, 1 out]
